vi "Asylum_StopPISLoop.vi"(8 "error in (no error)":errorcluster, 10 "whichLoop":i32, 11 "Application":refnum<k7>) -> (0 "error out":errorcluster, 3 "Application":refnum<k7>)   [LabVIEW 2019]
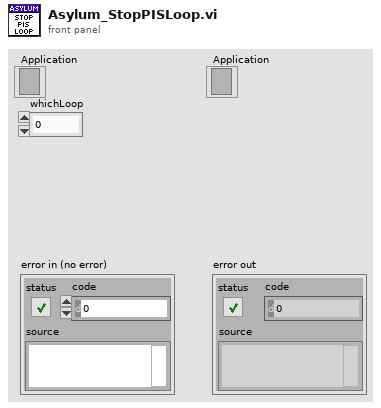
[diagram p1: front panel]
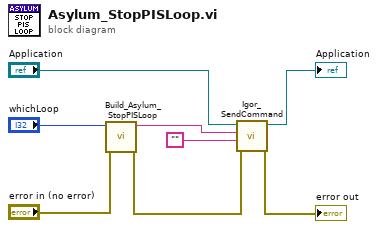
[diagram p0: block diagram]
diagram:
  n1 = call "Build_Asylum_StopPISLoop.vi"("error in (no error)"="error in (no error)", "whichLoop"="whichLoop") -> ("error out"=w8:errorcluster, "Command"=w6:string)  [unwired: 8 in]
  n2 = call "Igor_SendCommand.vi"("error in (no error)"=w8, "Format"="", "command"=w6, "Application In"="Application") -> ("error out"=→"error out":errorcluster, "Application Out"=→"Application":refnum<k7>)  [unwired: 4 in, 2 out]
